vi "ConvertPixelsToum.vi"(6 "error in (no error)":errorcluster, 8 "Parameters":T1={"number of planes"=4, "z step"=1.9999999999999998e-05, "pixel dwell time"=1.0000000000000001e-11, "z frequency"=10.0, "number of pixels"=100, "smooth points"=10, "smooth line"=10, "Sine\nSawtooth"=FALSE, "PointSorting"=0, "Sort Points"=FALSE, "X-pixels"=256.0, "Y-lines"=256.0, "pixelstoµm"=256.0, "zoom"=1.0, "Time offset"=1.0000000000000001e-11} {"zoom" min=0.5 step=0.1; "Y-lines" min=1 step=1; "X-pixels" min=1 step=1; "PointSorting" items=["No Difference", "Every Second Point", "Down / Up"]; "smooth line" min=1; "smooth points" min=1; "number of pixels" min=1; "z frequency" format="%_4g"; "number of planes" min=1}, 9 "Point coordinates (pixels)":dbl[][](array[numeric])) -> (0 "error out":errorcluster, 3 "Point coordinates (µm)":dbl[][](array[numeric]))   [LabVIEW 2010]
uses:
  TypeDefs/ParameterCluster.ctl
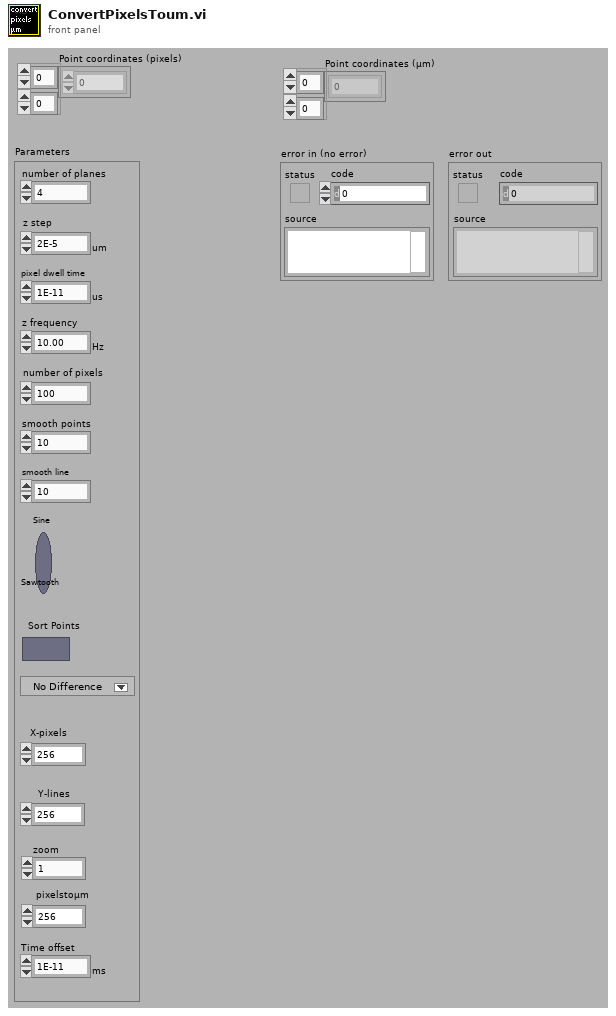
[diagram p1: front panel]
types:
  T1 = typedef "ParameterCluster.ctl" = cluster{"number of planes":i32, "z step":dbl[unit], "pixel dwell time":dbl[unit], "z frequency":dbl[unit], "number of pixels":i32, "smooth points":i32, "smooth line":i32, "Sine\nSawtooth":bool, "PointSorting":u16, "Sort Points":bool, "X-pixels":sgl, "Y-lines":sgl, "pixelstoµm":dbl, "zoom":dbl, "Time offset":dbl[unit]}
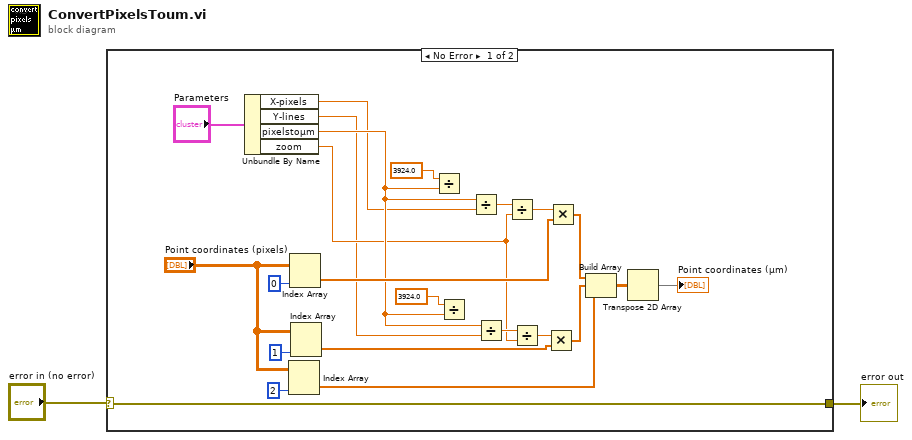
[diagram p0: block diagram]
diagram:
  n1 = case shown="No Error" "error in (no error)" {
    selector: "error in (no error)" -> [w6 w26]
    tunnel: [w6 w26] -> w1
    frame No Error {
      n2 = Unbundle By Name("Parameters") -> ("X-pixels"=w8:sgl, "Y-lines"=w7:sgl, "pixelstoµm"=w10:dbl, "zoom"=w9:dbl)
      n3 = Index Array(array="Point coordinates (pixels)", index (col)=2 ("disabled index (col)")) -> (element=w3:dbl[])  [unwired: 1 in]
      n4 = Index Array(array="Point coordinates (pixels)", index (col)=0 ("disabled index (col)")) -> (element=w20:dbl[])  [unwired: 1 in]
      n5 = Index Array(array="Point coordinates (pixels)", index (col)=1 ("disabled index (col)")) -> (element=w16:dbl[])  [unwired: 1 in]
      n6 = Divide(x=sgl 3924.0, y=w10) -> ()  [unwired: 1 out]
      n7 = Divide(x=sgl 3924.0, y=w10) -> ()  [unwired: 1 out]
      n8 = Divide(x=w10, y=w8) -> (x/y=w25:dbl)
      n9 = Divide(x=w10, y=w7) -> (x/y=w19:dbl)
      n10 = Divide(x=w25, y=w9) -> (x/y=w23:dbl)
      n11 = Divide(x=w19, y=w9) -> (x/y=w17:dbl)
      n12 = Multiply(x=w17, y=w16) -> (x*y=w13:dbl[])
      n13 = Multiply(x=w23, y=w20) -> (x*y=w14:dbl[])
      n14 = Build Array(w14, w13, w3) -> (w15:dbl[][])
      n15 = Transpose 2D Array(2D array=w15) -> (transposed array=→"Point coordinates (µm)":dbl[][])
    }
    frame Error {
    }
  }
  "error out" <- w1
